vi "Efficiency.vi"() -> ()   [LabVIEW 2021]
doc: "Demonstrates how to use triggers and events to synchronize multiple channels in Sequence source mode. Use this example to sequence multiple channels in lock-step."
uses:
  <instrlib>/niDCPower/nidcpower.llb/niDCPower Output Function.ctl
  <instrlib>/niDCPower/nidcpower.llb/niDCPower Source Mode.ctl
  <instrlib>/niDCPower/nidcpower.llb/niDCPower Sequence Attribute Type.ctl
  <instrlib>/niDCPower/nidcpower.llb/niDCPower Sense.ctl
  <instrlib>/niDCPower/nidcpower.llb/niDCPower Wait For Event - Event.ctl
  <vilib>/Analysis/1siggen.llb/Ramp Pattern by Samples.vi
  <instrlib>/niDCPower/nidcpower.llb/niDCPower Create Advanced Sequence Step.vi
  <instrlib>/niDCPower/nidcpower.llb/niDCPower Configure Digital Edge Source Trigger.vi
  <instrlib>/niDCPower/nidcpower.llb/niDCPower Configure Digital Edge Measure Trigger.vi
  <vilib>/Utility/file.llb/Write Delimited Spreadsheet (string).vi
  <vilib>/Utility/file.llb/Write Delimited Spreadsheet (DBL).vi
  <vilib>/Analysis/NI_AALBase.lvlib
panel:
  in  "Tab Control":enum32{"Main", "Debug"}(tab)
  in  "DUT setup time (s)":dbl=1.0 format="%.2p"
  in  "Source device name":refnum<k15>="PXI2Slot2"
  in  "Source device channel":string="0"
  in  "Source device max. power (W)":dbl=300.0
  in  "Source values (V)":dbl[](array[numeric])=[5.0, 10.0, 15.0, 20.0]
  in  "Source device max. current (A)":dbl=25.0
  in  "Current load level start":dbl=0.01 min=0.0 step=0.1
  in  "Current load level stop":dbl=2.5 min=0.0 step=0.1
  in  "Points or Points/Decade":i32=10 min=1
  in  "Load device channel":string="0"
  in  "Load device voltage limit (V)":dbl=5.0
  in  "Load device name":refnum<k15>="PXI2Slot4"
  in  "Timeout (s)":dbl=45.0 format="%.3p"
  in  "Sweep type":u16(ring)=1 items=["Linear", "Logarithmic"]
  in  "Aperture time (s)":dbl=0.1
  in  "Source delay (s)":dbl=0.1
  in  "Source device wait (s)":dbl=0.1
  out "DUT Efficiency (%) vs. Load Current (A)":cluster{dbl[], dbl[]}[](graph) caption="Current (Amps) vs Voltage (Volts)"
  out "Load Power":T1(graph) caption="Current (Amps) vs Voltage (Volts)"
  out "Supply Power":T1(graph) caption="Current (Amps) vs Voltage (Volts)"
  out "Load Current":T1(graph) caption="Current (Amps) vs Voltage (Volts)"
  out "Load Voltage":cluster{dbl[], "voltage measurements":dbl[]}(graph) caption="Current (Amps) vs Voltage (Volts)"
  out "Supply Current":T1(graph) caption="Current (Amps) vs Voltage (Volts)"
  out "Supply Voltage":T2(graph) caption="Current (Amps) vs Voltage (Volts)"
  in  "Export debug curves?":enum16{"No", "Yes"}(ring)
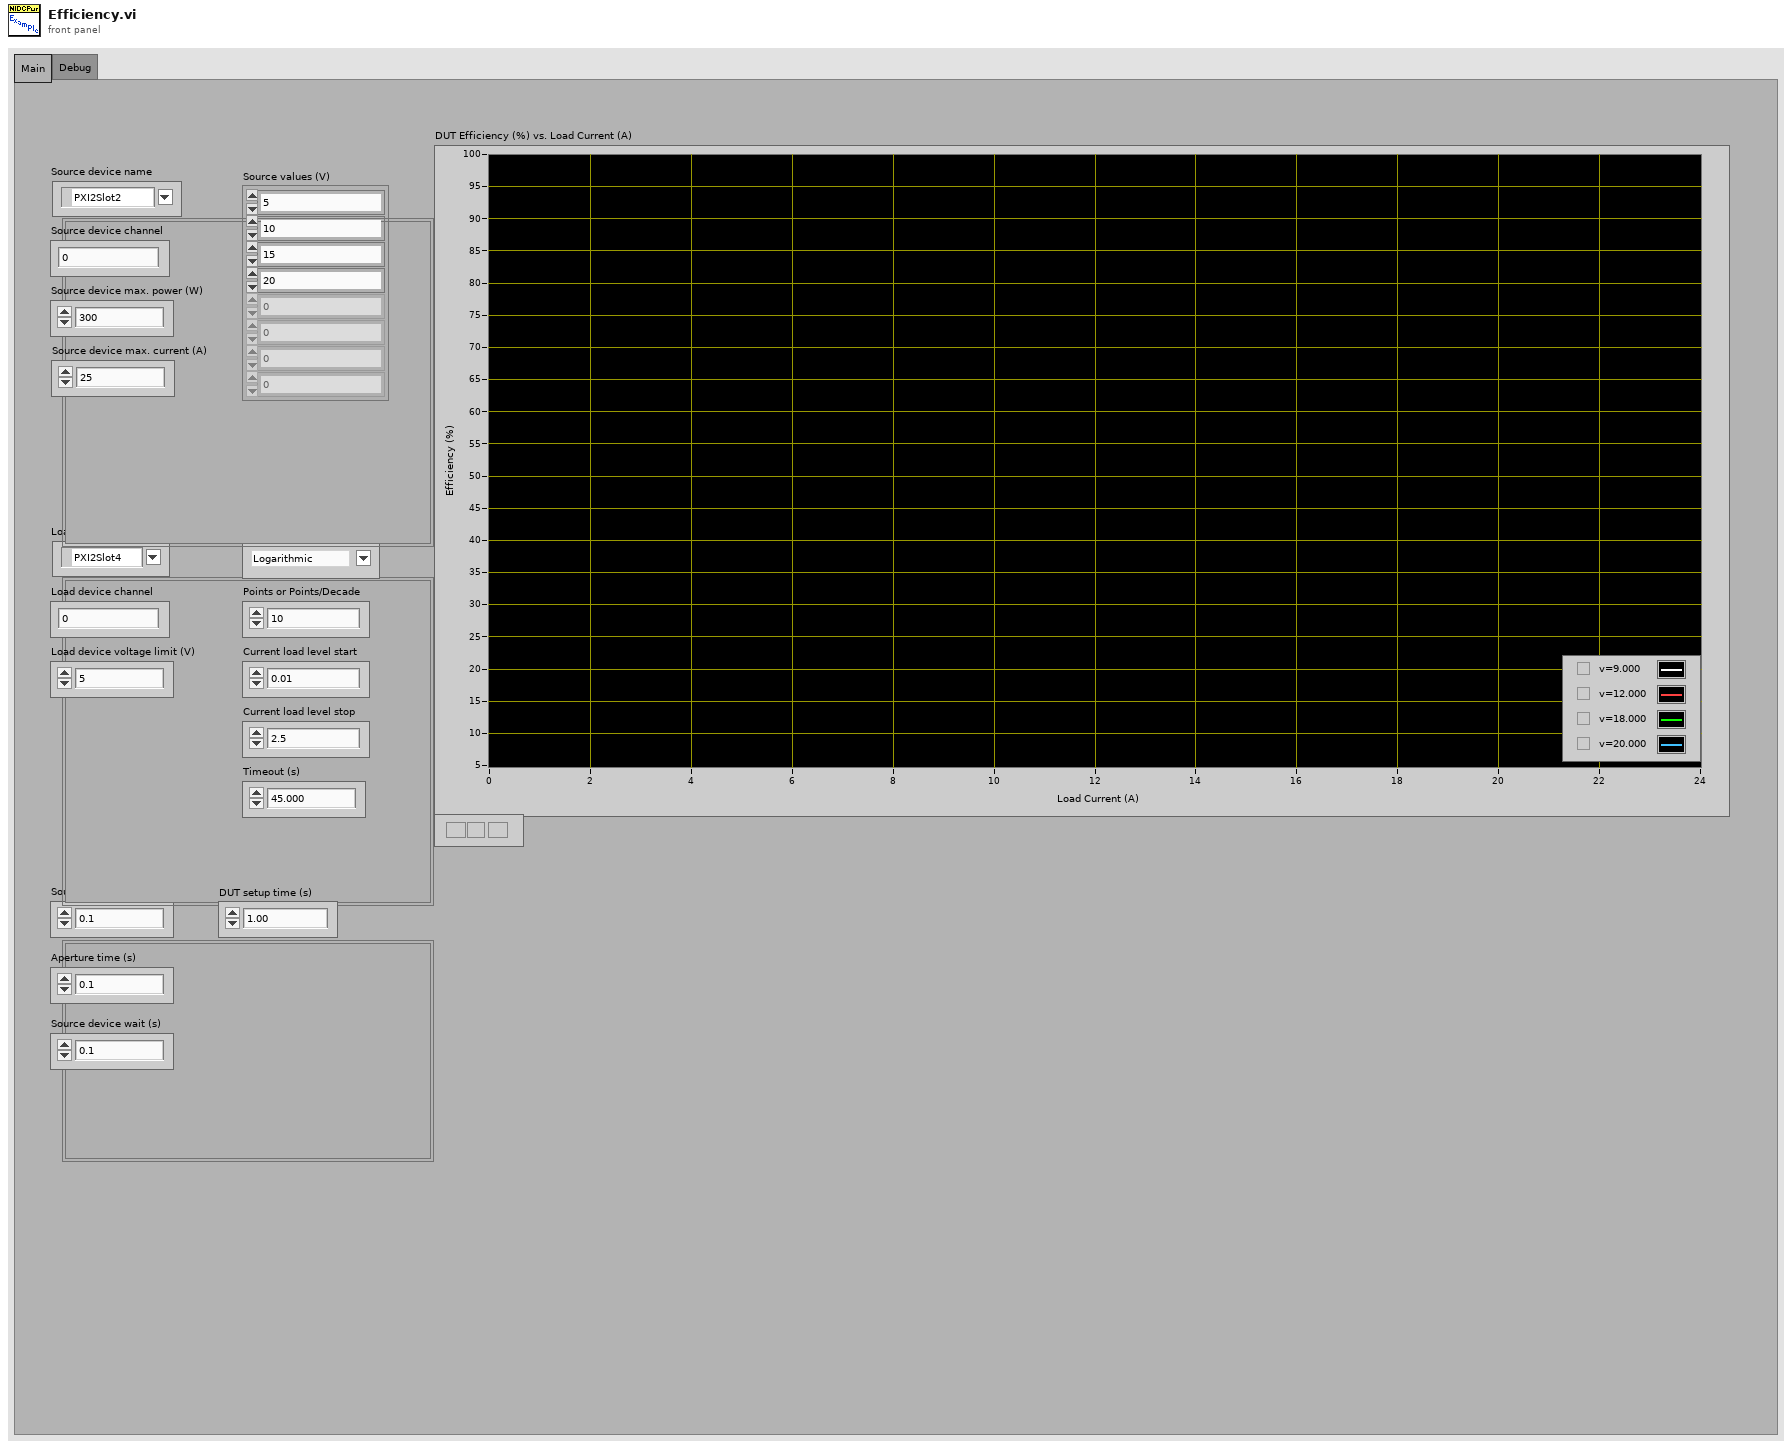
[diagram p1: front panel]
types:
  T1 = cluster{"Ramp Pattern":dbl[], "current measurements":dbl[]}
  T2 = cluster{"Ramp Pattern":dbl[], "voltage measurements":dbl[]}
  T3 = typedef "niDCPower Source Mode.ctl" = i32
  T4 = typedef "niDCPower Wait For Event - Event.ctl" = i32
  T5 = typedef "niDCPower Sense.ctl" = i32
  T6 = typedef "niDCPower Sequence Attribute Type.ctl" = i32
  T7 = typedef "niDCPower Output Function.ctl" = i32
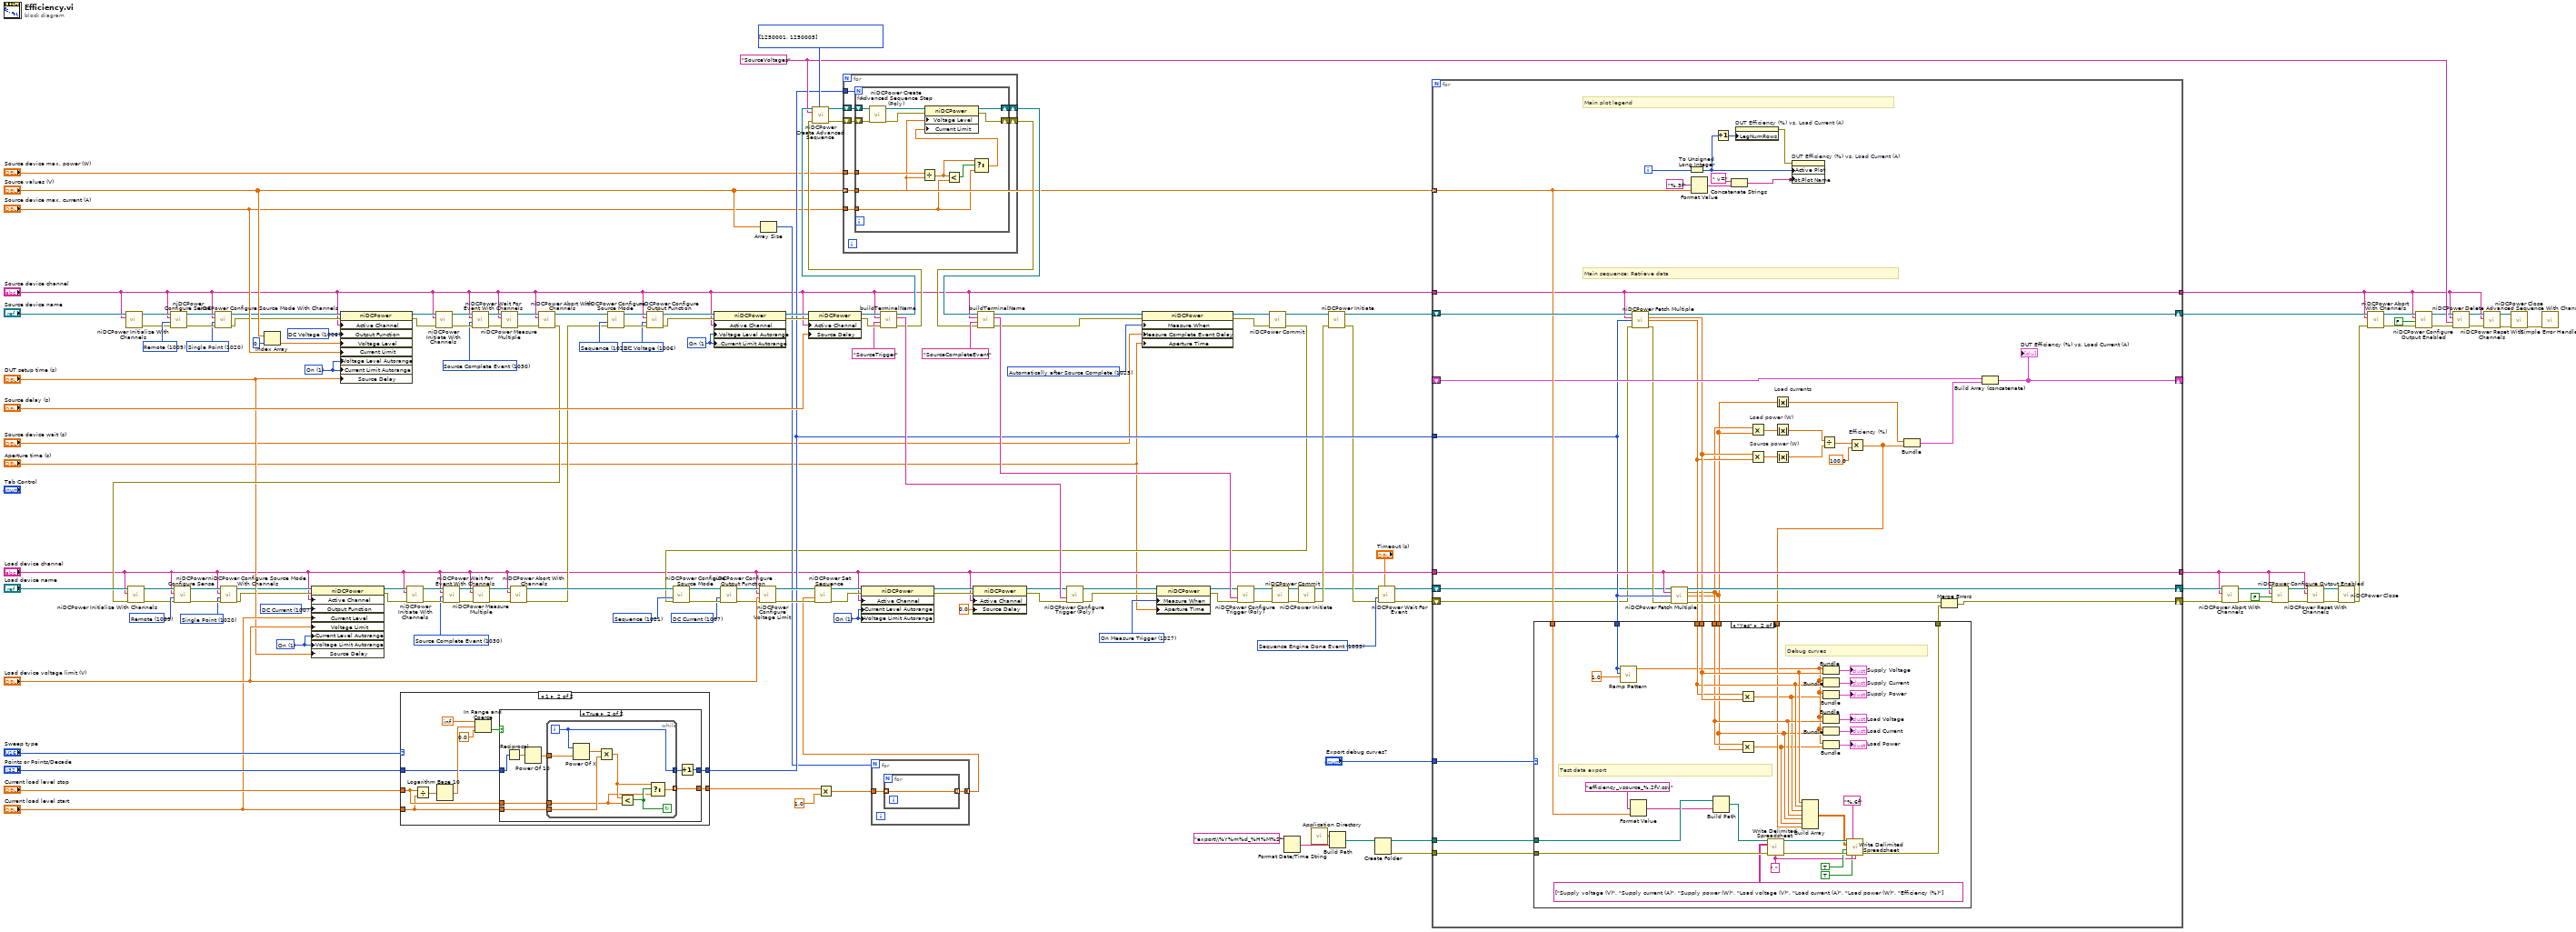
[diagram p0: block diagram]
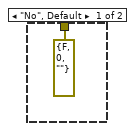
[diagram p2: hidden frame]
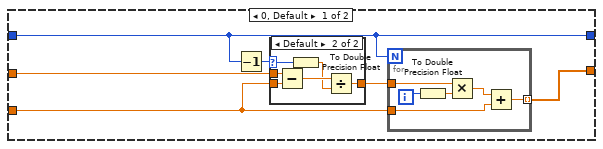
[diagram p3: hidden frame]
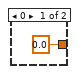
[diagram p4: hidden frame]
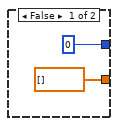
[diagram p5: hidden frame]
diagram:
  w28 = T3 1020 items=["Single Point"=1020, "Sequence"=1021] ("source mode")
  w35 = T3 1020 items=["Single Point"=1020, "Sequence"=1021] ("source mode")
  w41 = 1006 items=["DC Voltage"=1006, "DC Current"=1007, "Pulse Voltage"=1049, "Pulse Current"=1050] ("Source:Output Function")
  w58 = T4 1030 items=["Source Complete Event"=1030, "Measure Complete Event"=1031, "Sequence Iteration Complete Event"=1032, "Sequence Engine Done Event"=1033, "Pulse Complete Event"=1051, "Ready For Pulse Trigger Event"=1052] ("event")
  w63 = 1 items=["Off", "On"] ("Source:DC Current:Current Level Autorange")
  w72 = T4 1030 items=["Source Complete Event"=1030, "Measure Complete Event"=1031, "Sequence Iteration Complete Event"=1032, "Sequence Engine Done Event"=1033, "Pulse Complete Event"=1051, "Ready For Pulse Trigger Event"=1052] ("event")
  w82 = 1 items=["Off", "On"] ("Source:DC Current:Current Level Autorange")
  w83 = 1007 items=["DC Voltage"=1006, "DC Current"=1007, "Pulse Voltage"=1049, "Pulse Current"=1050] ("Source:Output Function")
  w91 = T5 1009 items=["Local"=1008, "Remote"=1009] ("sense")
  w11 = T4 1033 items=["Source Complete Event"=1030, "Measure Complete Event"=1031, "Sequence Iteration Complete Event"=1032, "Sequence Engine Done Event"=1033] ("event")
  w115 = 1 items=["Off", "On"] ("DC Voltage:Voltage Level Autorange")
  w116 = T5 1009 items=["Local"=1008, "Remote"=1009] ("sense")
  w130 = 1 items=["Off", "On"] ("DC Voltage:Voltage Level Autorange")
  w131 = T6[] [1250001, 1250005] items=["Source -> Output Function"=1150008, "Source -> Output Enabled"=1250006, "Source -> Output Resistance"=1150061, "Source -> Transient Response"=1150062, "Source -> Custom Transient Response -> Voltage Gain Bandwidth"=1150067, "Source -> Custom Transient Response -> Voltage Compensation Frequency"=1150068, "Source -> Custom Transient Response -> Voltage Pole-Zero Ratio"=1150069, "Source -> Custom Transient Response -> Current Gain Bandwidth"=1150070, "Source -> Custom Transient Response -> Current Compensation Frequency"=1150071, "Source -> Custom Transient Response -> Current Pole-Zero Ratio"=1150072, "Source -> DC Voltage -> Voltage Level"=1250001, "Source -> DC Voltage -> Voltage Level Range"=1150005, "Source -> DC Voltage -> Current Limit"=1250005, "Source -> DC Voltage -> Current Limit High"=1150187, "Source -> DC Voltage -> Current Limit Low"=1150188, "Source -> DC Voltage -> Current Limit Range"=1150004, "Source -> DC Current -> Current Level"=1150009, "Source -> DC Current -> Current Level Range"=1150011, "Source -> DC Current -> Voltage Limit"=1150010, "Source -> DC Current -> Voltage Limit High"=1150185, "Source -> DC Current -> Voltage Limit Low"=1150186, "Source -> DC Current -> Voltage Limit Range"=1150012, "Source -> Pulse Voltage -> Pulse Voltage Level"=1150080, "Source -> Pulse Voltage -> Pulse Bias Voltage Level"=1150082, "Source -> Pulse Voltage -> Pulse Voltage Level Range"=1150084, "Source -> Pulse Voltage -> Pulse Current Limit"=1150081, "Source -> Pulse Voltage -> Pulse Current Limit High"=1150193, "Source -> Pulse Voltage -> Pulse Current Limit Low"=1150194, "Source -> Pulse Voltage -> Pulse Bias Current Limit"=1150083, "Source -> Pulse Voltage -> Pulse Bias Current Limit High"=1150195, "Source -> Pulse Voltage -> Pulse Bias Current Limit Low"=1150196, "Source -> Pulse Voltage -> Pulse Current Limit Range"=1150085, "Source -> Pulse Current -> Pulse Current Level"=1150086, "Source -> Pulse Current -> Pulse Bias Current Level"=1150088, "Source -> Pulse Current -> Pulse Current Level Range"=1150090, "Source -> Pulse Current -> Pulse Voltage Limit"=1150087, "Source -> Pulse Current -> Pulse Voltage Limit High"=1150189, "Source -> Pulse Current -> Pulse Voltage Limit Low"=1150190, "Source -> Pulse Current -> Pulse Bias Voltage Limit"=1150089, "Source -> Pulse Current -> Pulse Bias Voltage Limit High"=1150191, "Source -> Pulse Current -> Pulse Bias Voltage Limit Low"=1150192, "Source -> Pulse Current -> Pulse Voltage Limit Range"=1150091, "Source -> Advanced -> Source Delay"=1150051, "Source -> Advanced -> Pulse Bias Delay"=1150092, "Source -> Advanced -> Pulse On Time"=1150093, "Source -> Advanced -> Pulse Off Time"=1150094, "Source -> Advanced -> OVP Enabled"=1250002, "Source -> Advanced -> OVP Limit"=1250003, "Source -> Advanced -> Compliance Limit Symmetry"=1150184, "Source -> Advanced -> Sequence Step Delta Time"=1150198, "Measurement -> Sense"=1150013, "Measurement -> Aperture Time"=1150058, "Measurement -> Measure Record Length"=1150063, "Measurement -> Advanced -> DC Noise Rejection"=1150066, "Measurement -> Autorange"=1150244, "Measurement -> Advanced -> Autorange Behavior"=1150245, "Measurement -> Advanced -> Autorange Aperture Time Mode"=1150246, "Measurement -> Advanced -> Autorange Minimum Aperture Time"=1150247, "Measurement -> Advanced -> Autorange Minimum Aperture Time Units"=1150248, "Measurement -> Advanced -> Autorange Minimum Current Range"=1150255, "Measurement -> Advanced -> Autorange Minimum Voltage Range"=1150256, "Measurement -> Advanced -> Autorange Threshold Mode"=1150257, "Measurement -> Advanced -> Autorange Maximum Delay After Range Change"=1150322, "LCR -> Instrument Mode"=1150208, "LCR -> LCR Stimulus Function"=1150209, "LCR -> LCR Frequency"=1150210, "LCR -> LCR Voltage Amplitude"=1150211, "LCR -> LCR Current Amplitude"=1150212, "LCR -> LCR DC Bias Source"=1150213, "LCR -> LCR DC Bias Voltage Level"=1150214, "LCR -> LCR DC Bias Current Level"=1150215, "LCR -> LCR Impedance Autorange"=1150216, "LCR -> LCR Impedance Range"=1150217, "LCR -> LCR Measurement Time"=1150218, "LCR -> LCR Custom Measurement Time"=1150258, "LCR -> LCR Source Delay Mode"=1150315, "LCR -> Compensation -> Open -> Enabled"=1150220, "LCR -> Compensation -> Open -> Conductance"=1150261, "LCR -> Compensation -> Open -> Susceptance"=1150262, "LCR -> Compensation -> Short -> Enabled"=1150221, "LCR -> Compensation -> Short -> Resistance"=1150263, "LCR -> Compensation -> Short -> Reactance"=1150264, "LCR -> Compensation -> Load -> Enabled"=1150222, "LCR -> Compensation -> Load -> Measured Resistance"=1150268, "LCR -> Compensation -> Load -> Measured Reactance"=1150269, "LCR -> Compensation -> Load -> Actual Resistance"=1150270, "LCR -> Compensation -> Load -> Actual Reactance"=1150271] ("advanced sequence properties")
  w104 = "SourceVoltages" ("sequence name")
  w136 = T7 1007 items=["DC Voltage"=1006, "DC Current"=1007, "Pulse Voltage"=1049, "Pulse Current"=1050] ("output function")
  w137 = 1027 items=["Automatically after Source Complete"=1025, "On Demand"=1026, "On Measure Trigger"=1027] ("Measurement:Advanced:Measure When")
  w138 = T3 1021 items=["Single Point"=1020, "Sequence"=1021] ("source mode")
  w145 = T7 1006 items=["DC Voltage"=1006, "DC Current"=1007, "Pulse Voltage"=1049, "Pulse Current"=1050] ("output function")
  w4 = 1025 items=["Automatically after Source Complete"=1025, "On Demand"=1026, "On Measure Trigger"=1027] ("Measurement:Advanced:Measure When")
  w155 = T3 1021 items=["Single Point"=1020, "Sequence"=1021] ("source mode")
  n1 = call <instrlib>:"niDCPower Initialize With Channels.vi"("channels"="Source device channel", "resource name"="Source device name") -> ("error out"=w66:errorcluster, "instrument handle out"=w67:refnum<k15>)  [unwired: 3 in, 5 out]
  n2 = call <instrlib>:"niDCPower Configure Sense.vi"("error in (no error)"=w66, "sense"=w91, "channel name"="Source device channel", "instrument handle"=w67) -> ("error out"=w38:errorcluster, "instrument handle out"=w40:refnum<k15>)  [unwired: 6 in]
  n3 = call <instrlib>:"niDCPower Configure Source Mode With Channels.vi"("error in (no error)"=w38, "source mode"=w35, "channel name"="Source device channel", "instrument handle"=w40) -> ("error out"=w37:errorcluster, "instrument handle out"=w39:refnum<k15>)  [unwired: 6 in]
  n4 = Index Array(array="Source values (V)", index=0) -> (element=w52:dbl)
  n5 = property class="niDCPower"(reference=w39, error in=w37, "Active Channel"="Source device channel", "Output Function"=w41, "Voltage Level"=w52, "Current Limit"="Source device max. current (A)", "Voltage Level Autorange"=w63, "Current Limit Autorange"=w63, "Source Delay"="DUT setup time (s)") -> (reference out=w61:refnum<k15>, error out=w62:errorcluster)
  n6 = case shown="1" "Sweep type" {
    tunnel: "Points or Points/Decade" -> [w160 w179]
    tunnel: [w163 w183] -> w121
    tunnel: "Current load level start" -> [w162 w180]
    tunnel: "Current load level stop" -> [w161 w187]
    tunnel: [w160 w184] -> w103
    frame 0, Default {
      n7 = Decrement(x=w160) -> (x-1=w165:i32)
      n8 = case shown="Default" w165 {
        selector: w165 -> [_ w173]
        tunnel: w161 -> [_ w178]
        tunnel: w162 -> [_ w177]
        tunnel: [0.0 w175] -> w164
        frame 0 {
        }
        frame Default {
          n9 = Subtract(x=w178, y=w177) -> (x-y=w176:dbl)
          n10 = To Double Precision Float(number=w173) -> (double precision float=w174:dbl)
          n11 = Divide(x=w176, y=w174) -> (x/y=w175:dbl)
        }
      }
      n12 = for {
        N: w160 -> [_]
        tunnel: w164 -> [w170]
        tunnel: w162 -> [w171]
        tunnel: [w166] -> w163 mode=indexing
        i -> [w169]
        n13 = To Double Precision Float(number=w169) -> (double precision float=w167:dbl)
        n14 = Multiply(x=w170, y=w167) -> (x*y=w168:dbl)
        n15 = Add(x=w168, y=w171) -> (x+y=w166:dbl)
      }
    }
    frame 1 {
      n16 = Divide(x=w187, y=w180) -> (x/y=w188:dbl)
      n17 = Logarithm Base 10(1:w188) -> (0:w185:dbl)
      n18 = In Range and Coerce(upper limit=inf, x=w185, lower limit=0.0) -> (In Range?=w182:bool)  [unwired: 1 out]
      n19 = case shown="True" w182 {
        tunnel: [dbl[] [] w198] -> w183
        tunnel: [0 w191] -> w184
        tunnel: w187 -> [_ w197]
        tunnel: w180 -> [_ w196]
        tunnel: w179 -> [_ w193]
        frame False {
        }
        frame True {
          n20 = Reciprocal(x=w193) -> (1/x=w195:dbl)
          n21 = Power Of 10(x=w195) -> (10^x=w194:dbl)
          n22 = while {
            tunnel: w194 -> [w203]
            tunnel: w196 -> [w206]
            tunnel: [w202] -> w198 mode=indexing
            tunnel: [w204] -> w192
            tunnel: w197 -> [w199]
            i -> [w204]
            stop <- w201 continue-if-true
            n23 = Power Of X(1:w203, 2:w204) -> (0:w205:dbl)
            n24 = Multiply(x=w205, y=w206) -> (x*y=w200:dbl)
            n25 = Less?(x=w200, y=w199) -> (x < y?=w201:bool)
            n26 = Select(t=w200, s=w201, f=w199) -> (s? t:f=w202:dbl)
          }
          n27 = Increment(x=w192) -> (x+1=w191:i32)
        }
      }
    }
  }
  n28 = call <instrlib>:"niDCPower Initiate With Channels.vi"("error in (no error)"=w62, "channel name"="Source device channel", "instrument handle"=w61) -> ("error out"=w60:errorcluster, "instrument handle out"=w59:refnum<k15>)  [unwired: 7 in]
  n29 = call <instrlib>:"niDCPower Wait For Event With Channels.vi"("error in (no error)"=w60, "event"=w58, "channel name"="Source device channel", "instrument handle"=w59) -> ("error out"=w57:errorcluster, "instrument handle out"=w56:refnum<k15>)  [unwired: 6 in]
  n30 = call <instrlib>:"niDCPower Measure Multiple.vi"("error in (no error)"=w57, "channel name"="Source device channel", "instrument handle"=w56) -> ("error out"=w54:errorcluster, "instrument handle out"=w55:refnum<k15>)  [unwired: 5 in, 2 out]
  n31 = call <instrlib>:"niDCPower Abort With Channels.vi"("error in (no error)"=w54, "channel name"="Source device channel", "instrument handle"=w55) -> ("error out"=w48:errorcluster, "instrument handle out"=w49:refnum<k15>)  [unwired: 7 in]
  n32 = call <instrlib>:"niDCPower Initialize With Channels.vi"("error in (no error)"=w48, "channels"="Load device channel", "resource name"="Load device name") -> ("error out"=w80:errorcluster, "instrument handle out"=w81:refnum<k15>)  [unwired: 2 in, 5 out]
  n33 = call <instrlib>:"niDCPower Configure Sense.vi"("error in (no error)"=w80, "sense"=w116, "channel name"="Load device channel", "instrument handle"=w81) -> ("error out"=w32:errorcluster, "instrument handle out"=w33:refnum<k15>)  [unwired: 6 in]
  n34 = call <instrlib>:"niDCPower Configure Source Mode With Channels.vi"("error in (no error)"=w32, "source mode"=w28, "channel name"="Load device channel", "instrument handle"=w33) -> ("error out"=w30:errorcluster, "instrument handle out"=w31:refnum<k15>)  [unwired: 6 in]
  n35 = property class="niDCPower"(reference=w31, error in=w30, "Active Channel"="Load device channel", "Output Function"=w83, "Current Level"="Current load level start", "Voltage Limit"="Load device voltage limit (V)", "Current Level Autorange"=w82, "Voltage Limit Autorange"=w82, "Source Delay"="DUT setup time (s)") -> (reference out=w75:refnum<k15>, error out=w76:errorcluster)
  n36 = call <instrlib>:"niDCPower Initiate With Channels.vi"("error in (no error)"=w76, "channel name"="Load device channel", "instrument handle"=w75) -> ("error out"=w74:errorcluster, "instrument handle out"=w73:refnum<k15>)  [unwired: 7 in]
  n37 = call <instrlib>:"niDCPower Wait For Event With Channels.vi"("error in (no error)"=w74, "event"=w72, "channel name"="Load device channel", "instrument handle"=w73) -> ("error out"=w71:errorcluster, "instrument handle out"=w70:refnum<k15>)  [unwired: 6 in]
  n38 = call <instrlib>:"niDCPower Measure Multiple.vi"("error in (no error)"=w71, "channel name"="Load device channel", "instrument handle"=w70) -> ("error out"=w68:errorcluster, "instrument handle out"=w69:refnum<k15>)  [unwired: 5 in, 2 out]
  n39 = call <instrlib>:"niDCPower Abort With Channels.vi"("error in (no error)"=w68, "channel name"="Load device channel", "instrument handle"=w69) -> ("error out"=w46:errorcluster, "instrument handle out"=w47:refnum<k15>)  [unwired: 7 in]
  n40 = call <instrlib>:"niDCPower Configure Source Mode.vi"("error in (no error)"=w46, "source mode"=w155, "instrument handle"=w49) -> ("error out"=w157:errorcluster, "instrument handle out"=w156:refnum<k15>)  [unwired: 7 out]
  n41 = call <instrlib>:"niDCPower Configure Output Function.vi"("error in (no error)"=w157, "output function"=w145, "channel name"="Source device channel", "instrument handle"=w156) -> ("error out"=w64:errorcluster, "instrument handle out"=w65:refnum<k15>)  [unwired: 6 out]
  n42 = property class="niDCPower"(reference=w65, error in=w64, "Active Channel"="Source device channel", "Source:DC Voltage:Voltage Level Autorange"=w130, "Source:DC Voltage:Current Limit Autorange"=w130) -> (reference out=w128:refnum<k15>, error out=w127:errorcluster)
  n43 = Array Size(array="Source values (V)") -> (size(s)=w96:i32)
  n44 = property class="niDCPower"(reference=w128, error in=w127, "Active Channel"="Source device channel", "Source Delay"="Source delay (s)") -> (reference out=w151:refnum<k15>, error out=w150:errorcluster)
  n45 = Multiply(x=w121, y=1.0) -> (x*y=w98:dbl[])
  n46 = for {
    N: w96 -> [_]
    tunnel: w98 -> [w208]
    tunnel: [w207] -> w97 mode=concatenating
    n47 = for {
      tunnel: w208 -> [w209] mode=indexing
      tunnel: [w209] -> w207 mode=indexing
    }
  }
  n48 = call "buildTerminalName.vi"("error in (no error)"=w150, "Local Terminal Name"="SourceTrigger", "Channel Name"="Source device channel", "session handle"=w151) -> ("error IO"=w123:errorcluster, "Fully Qualified Terminal Name"=w148:string, "session handle 2"=w125:refnum<k15>)  [unwired: 5 out]
  n49 = call <instrlib>:"niDCPower Create Advanced Sequence.vi"("instrument handle"=w125, "sequence name"=w104, "advanced sequence properties"=w131, "error in (no error)"=w123) -> ("instrument handle out"=w133:refnum<k15>, "error out"=w132:errorcluster)  [unwired: 10 in]
  n50 = for {
    tunnel: "Source device max. power (W)" -> [w213]
    tunnel: "Source device max. current (A)" -> [w212]
    tunnel: "Source values (V)" -> [w211] mode=indexing
    shift-right: [w215] -> w124
    shift-left: w133 -> [w217]
    shift-right: [w214] -> w122
    shift-left: w132 -> [w216]
    tunnel: w103 -> [w210]
    n51 = for {
      N: w210 -> [_]
      shift-right: [w226] -> w214
      shift-left: w216 -> [w229]
      shift-right: [w225] -> w215
      shift-left: w217 -> [w224]
      tunnel: w213 -> [w223]
      tunnel: w211 -> [w218]
      tunnel: w212 -> [w221]
      n52 = call-poly <instrlib>:"niDCPower Create Advanced Sequence Step (Poly).vi"("error in (no error)"=w229, "instrument handle"=w224) -> ("error out"=w227:errorcluster, "instrument handle out"=w228:refnum<k15>)  [unwired: 8 in]
      n53 = Divide(x=w223, y=w218) -> (x/y=w220:dbl)
      n54 = Less?(x=w220, y=w221) -> (x < y?=w222:bool)
      n55 = Select(t=w220, s=w222, f=w221) -> (s? t:f=w219:dbl)
      n56 = property class="niDCPower"(reference=w228, error in=w227, "Voltage Level"=w218, "Current Limit"=w219) -> (reference out=w225:refnum<k15>, error out=w226:errorcluster)
    }
  }
  n57 = call "buildTerminalName.vi"("error in (no error)"=w122, "Local Terminal Name"="SourceCompleteEvent", "Channel Name"="Source device channel", "session handle"=w124) -> ("error IO"=w2:errorcluster, "Fully Qualified Terminal Name"=w147:string, "session handle 2"=w3:refnum<k15>)  [unwired: 5 out]
  n58 = property class="niDCPower"(reference=w3, error in=w2, "Measure When"=w4, "Measure Complete Event Delay"="Source device wait (s)", "Aperture Time"="Aperture time (s)") -> (reference out=w153:refnum<k15>, error out=w152:errorcluster)
  n59 = call <instrlib>:"niDCPower Commit.vi"("error in (no error)"=w152, "instrument handle"=w153) -> ("error out"=w45:errorcluster, "instrument handle out"=w93:refnum<k15>)  [unwired: 8 out]
  n60 = call <instrlib>:"niDCPower Configure Source Mode.vi"("error in (no error)"=w45, "source mode"=w138, "instrument handle"=w47) -> ("error out"=w140:errorcluster, "instrument handle out"=w139:refnum<k15>)  [unwired: 7 out]
  n61 = call <instrlib>:"niDCPower Configure Output Function.vi"("error in (no error)"=w140, "output function"=w136, "instrument handle"=w139) -> ("error out"=w43:errorcluster, "instrument handle out"=w44:refnum<k15>)  [unwired: 1 in, 6 out]
  n62 = call <instrlib>:"niDCPower Configure Voltage Limit.vi"("error in (no error)"=w43, "voltage limit"="Load device voltage limit (V)", "channel name"="Load device channel", "instrument handle"=w44) -> ("error out"=w111:errorcluster, "instrument handle out"=w112:refnum<k15>)  [unwired: 6 in]
  n63 = call <instrlib>:"niDCPower Set Sequence.vi"("error in (no error)"=w111, "values"=w97, "instrument handle"=w112) -> ("error out"=w99:errorcluster, "instrument handle out"=w100:refnum<k15>)  [unwired: 2 in, 5 out]
  n64 = property class="niDCPower"(reference=w100, error in=w99, "Active Channel"="Load device channel", "Current Level Autorange"=w115, "Voltage Limit Autorange"=w115) -> (reference out=w114:refnum<k15>, error out=w113:errorcluster)
  n65 = property class="niDCPower"(reference=w114, error in=w113, "Active Channel"="Load device channel", "Source Delay"=0.0 ("Source:Advanced:Source Delay")) -> (reference out=w102:refnum<k15>, error out=w101:errorcluster)
  n66 = call-poly <instrlib>:"niDCPower Configure Trigger (Poly).vi"("error in (no error)"=w101, "input terminal"=w148, "instrument handle"=w102) -> ("error out"=w143:errorcluster, "instrument handle out"=w144:refnum<k15>)  [unwired: 1 in, 6 out]
  n67 = property class="niDCPower"(reference=w144, error in=w143, "Measure When"=w137, "Aperture Time"="Aperture time (s)") -> (reference out=w141:refnum<k15>, error out=w142:errorcluster)
  n68 = call-poly <instrlib>:"niDCPower Configure Trigger (Poly).vi"("error in (no error)"=w142, "input terminal"=w147, "instrument handle"=w141) -> ("error out"=w95:errorcluster, "instrument handle out"=w94:refnum<k15>)  [unwired: 1 in, 6 out]
  n69 = call <instrlib>:"niDCPower Commit.vi"("error in (no error)"=w95, "instrument handle"=w94) -> ("error out"=w158:errorcluster, "instrument handle out"=w159:refnum<k15>)  [unwired: 8 out]
  n70 = Format Date/Time String(time format string (%c)="export\\%Y%m%d_%H%M%S") -> (date/time string=w87:string)  [unwired: 2 in]
  n71 = call <instrlib>:"niDCPower Initiate.vi"("error in (no error)"=w158, "instrument handle"=w159) -> ("error out"=w154:errorcluster, "instrument handle out"=w9:refnum<k15>)  [unwired: 8 out]
  n72 = call <vilib>:"Application Directory.vi"() -> ("Application Directory"=w88:path)
  n73 = call <instrlib>:"niDCPower Initiate.vi"("error in (no error)"=w154, "instrument handle"=w93) -> ("error out"=w10:errorcluster, "instrument handle out"=w110:refnum<k15>)  [unwired: 8 out]
  n74 = Build Path(base path=w88, name or relative path=w87) -> (appended path=w89:path)
  n75 = Create Folder(path (use dialog)=w89) -> (created path=w85:path, error out=w86:errorcluster)  [unwired: 2 in, 1 out]
  n76 = call <instrlib>:"niDCPower Wait For Event.vi"("timeout (10.0)"="Timeout (s)", "error in (no error)"=w10, "event"=w11, "instrument handle"=w9) -> ("error out"=w7:errorcluster, "instrument handle out"=w8:refnum<k15>)  [unwired: 6 out]
  n77 = for {
    tunnel: "Load device channel" -> [w259]
    tunnel: "Source device channel" -> [w258]
    shift-right: [w265] -> w84
    shift-left: w8 -> [w231]
    shift-right: [w263] -> w26
    shift-left: w7 -> [w230]
    shift-right: [w267] -> w105
    shift-left: w110 -> [w268]
    tunnel: w103 -> [w255]
    tunnel: "Source values (V)" -> [w264] mode=indexing
    tunnel: w86 -> [w262]
    tunnel: w85 -> [w261]
    tunnel: "Export debug curves?" -> [w260]
    tunnel: [w259] -> w12
    tunnel: [w258] -> w14
    shift-right: [w256] -> _
    shift-left: _ -> [w257]
    i -> [w266]
    # "Main sequence; Retrieve data"
    # "Main plot legend"
    n78 = call <instrlib>:"niDCPower Fetch Multiple.vi"("instrument handle"=w268, "channel name"=w258, "count (1)"=w255, "error in (no error)"=w230) -> ("instrument handle out"=w267:refnum<k15>, "voltage measurements"=w237:dbl[], "current measurements"=w236:dbl[], "error out"=w254:errorcluster)  [unwired: 1 in, 7 out]
    n79 = call <instrlib>:"niDCPower Fetch Multiple.vi"("instrument handle"=w231, "channel name"=w259, "count (1)"=w255, "error in (no error)"=w254) -> ("instrument handle out"=w265:refnum<k15>, "voltage measurements"=w235:dbl[], "current measurements"=w234:dbl[], "error out"=w239:errorcluster)  [unwired: 1 in, 7 out]
    n80 = To Unsigned Long Integer(number=w266) -> (unsigned 32bit integer=w250:u32)
    n81 = Format Value(format string="%.3f", value (0)=w264) -> (output string=w251:string)  [unwired: 1 out]
    n82 = Increment(x=w250) -> (x+1=w248:u32)
    n83 = Concatenate Strings(" v=" ("string"), w251) -> (w249:string)
    n84 = property on="DUT Efficiency (%) vs. Load Current (A)" class="XYGraph (strict)"("LegNumRows"=w248) -> (error out=w247:errorcluster)  [unwired: 2 in, 1 out]
    n85 = Multiply "Load power (W)"(x=w235, y=w234) -> (x*y=w245:dbl[])
    n86 = Multiply "Source power (W)"(x=w237, y=w236) -> (x*y=w244:dbl[])
    n87 = Absolute Value "Load currents"(x=w234) -> (abs(x)=w246:dbl[])
    n88 = Absolute Value(x=w245) -> (abs(x)=w242:dbl[])
    n89 = Absolute Value(x=w244) -> (abs(x)=w243:dbl[])
    n90 = property on="DUT Efficiency (%) vs. Load Current (A)" class="XYGraph (strict)"(error in=w247, "Active Plot"=w250, "Plot.Plot Name"=w249) -> ()  [unwired: 1 in, 2 out]
    n91 = Divide(x=w242, y=w243) -> (x/y=w241:dbl[])
    n92 = Multiply "Efficiency (%)"(x=w241, y=100.0) -> (x*y=w233:dbl[])
    n93 = case shown="\"Yes\"" w260 {
      tunnel: w255 -> [_ w300]
      tunnel: w264 -> [_ w299]
      tunnel: w262 -> [_ w298]
      tunnel: w261 -> [_ w297]
      tunnel: [errorcluster {"status"=FALSE, "code"=0, "source"=""} ("error out") w296] -> w238
      tunnel: w237 -> [_ w295]
      tunnel: w236 -> [_ w294]
      tunnel: w235 -> [_ w293]
      tunnel: w234 -> [_ w292]
      tunnel: w233 -> [_ w291]
      frame "No", Default {
      }
      frame "Yes" {
        w272 = "," ("delimiter (\\t)")
        # "Test data export"
        # "Debug curves"
        n94 = call-poly <vilib>:"Ramp Pattern.vi"("start"=1.0, "end"=w300, "samples"=w300) -> ("Ramp Pattern"=w283:dbl[])  [unwired: 7 in, 1 out]
        n95 = Format Value(format string="efficiency_vsource_%.2fV.csv" ("string"), value (0)=w299) -> (output string=w281:string)  [unwired: 1 out]
        n96 = Build Path(base path=w297, name or relative path=w281) -> (appended path=w280:path)
        n97 = Multiply(x=w294, y=w295) -> (x*y=w275:dbl[])
        n98 = Multiply(x=w293, y=w292) -> (x*y=w274:dbl[])
        n99 = call-poly <vilib>:"Write Delimited Spreadsheet.vi"("file path (dialog if empty)"=w280, "2D data"=string[][] [["Supply voltage (V)", "Supply current (A)", "Supply power (W)", "Load voltage (V)", "Load current (A)", "Load power (W)", "Efficiency (%)"]], "error in (no error)"=w298, "delimiter (\\t)"=w272) -> ("new file path (Not A Path if cancelled)"=w278:path, "error out"=w277:errorcluster)  [unwired: 10 in]
        n100 = Build Array(w295, w294, w275, w293, w292, w274, w291) -> (w273:dbl[][])
        n101 = Bundle("Ramp Pattern"=w283, "voltage measurements"=w295) -> (→"Supply Voltage":T2)  [unwired: 1 out]
        n102 = Bundle("Ramp Pattern"=w283, "current measurements"=w294) -> (→"Supply Current":T1)  [unwired: 1 out]
        n103 = Bundle("Ramp Pattern"=w283, w275) -> (→"Supply Power":cluster{"Ramp Pattern":dbl[], dbl[]})  [unwired: 1 out]
        n104 = Bundle("Ramp Pattern"=w283, "voltage measurements"=w293) -> (→"Load Voltage":T2)  [unwired: 1 out]
        n105 = Bundle("Ramp Pattern"=w283, "current measurements"=w292) -> (→"Load Current":T1)  [unwired: 1 out]
        n106 = Bundle("Ramp Pattern"=w283, w274) -> (→"Load Power":cluster{"Ramp Pattern":dbl[], dbl[]})  [unwired: 1 out]
        n107 = call-poly <vilib>:"Write Delimited Spreadsheet.vi"("file path (dialog if empty)"=w278, "format (%.3f)"="%.6f", "2D data"=w273, "append to file? (new file:F)"=TRUE, "error in (no error)"=w277, "transpose? (no:F)"=TRUE, "delimiter (\\t)"=w272) -> ("error out"=w296:errorcluster)  [unwired: 7 in, 1 out]
      }
    }
    n108 = Bundle(w246, w233) -> (w232:cluster{dbl[], dbl[]})  [unwired: 1 out]
    n109 = Merge Errors(w239, w238) -> (w263:errorcluster)
    n110 = Build Array (concatenate)(w257, w232) -> (w256:cluster{dbl[], dbl[]}[])
    "DUT Efficiency (%) vs. Load Current (A)" <- w256
  }
  n111 = call <instrlib>:"niDCPower Abort With Channels.vi"("error in (no error)"=w26, "channel name"=w12, "instrument handle"=w84) -> ("error out"=w24:errorcluster, "instrument handle out"=w25:refnum<k15>)  [unwired: 7 in]
  n112 = call <instrlib>:"niDCPower Configure Output Enabled.vi"("error in (no error)"=w24, "output enabled"=FALSE, "channel name"=w12, "instrument handle"=w25) -> ("error out"=w21:errorcluster, "instrument handle out"=w22:refnum<k15>)  [unwired: 6 in]
  n113 = call <instrlib>:"niDCPower Reset With Channels.vi"("error in (no error)"=w21, "channel name"=w12, "instrument handle"=w22) -> ("error out"=w135:errorcluster, "instrument handle out"=w134:refnum<k15>)  [unwired: 7 in]
  n114 = call <instrlib>:"niDCPower Close.vi"("error in (no error)"=w135, "instrument handle"=w134) -> ("error out"=w19:errorcluster)  [unwired: 9 out]
  n115 = call <instrlib>:"niDCPower Abort With Channels.vi"("error in (no error)"=w19, "channel name"=w14, "instrument handle"=w105) -> ("error out"=w18:errorcluster, "instrument handle out"=w17:refnum<k15>)  [unwired: 7 in]
  n116 = call <instrlib>:"niDCPower Configure Output Enabled.vi"("error in (no error)"=w18, "output enabled"=FALSE, "channel name"=w14, "instrument handle"=w17) -> ("error out"=w15:errorcluster, "instrument handle out"=w16:refnum<k15>)  [unwired: 6 in]
  n117 = call <instrlib>:"niDCPower Delete Advanced Sequence With Channels.vi"("error in (no error)"=w15, "sequence name"=w104, "channel name"=w14, "instrument handle"=w16) -> ("error out"=w106:errorcluster, "instrument handle out"=w107:refnum<k15>)  [unwired: 6 in]
  n118 = call <instrlib>:"niDCPower Reset With Channels.vi"("error in (no error)"=w106, "channel name"=w14, "instrument handle"=w107) -> ("error out"=w108:errorcluster, "instrument handle out"=w109:refnum<k15>)  [unwired: 7 in]
  n119 = call <instrlib>:"niDCPower Close.vi"("error in (no error)"=w108, "instrument handle"=w109) -> ("error out"=w20:errorcluster)  [unwired: 9 out]
  n120 = call <vilib>:"Simple Error Handler.vi"("error in (no error)"=w20) -> ()  [unwired: 1 in, 8 out]
